vi "Parse Xml Recursively.vi"(6 "Map in":map{string, T1}(c390), 7 "Parent":string, 8 "error in":errorcluster, 9 "XML File Path":path, 10 "DOM document in":refnum<k20>, 11 "Tree Map in":refnum<class "Tree Map.lvclass">) -> (0 "error out":errorcluster, 2 "Map out":map{string, T1}(c390), 3 "Tree Map out":refnum<class "Tree Map.lvclass">)   [LabVIEW 2023, in "VI Properties Editor.lvlib"]
uses:
  VI Properties Editor.lvlib
  Tree Map/Tree Map/Tree Map.lvclass
  CTLs/XPath Get Attribute.ctl
  <vilib>/picture/picture.llb/imagedata.ctl
  CTLs/VI Properties.ctl
  CTLs/Control Properties.ctl
  CTLs/VI Data.ctl
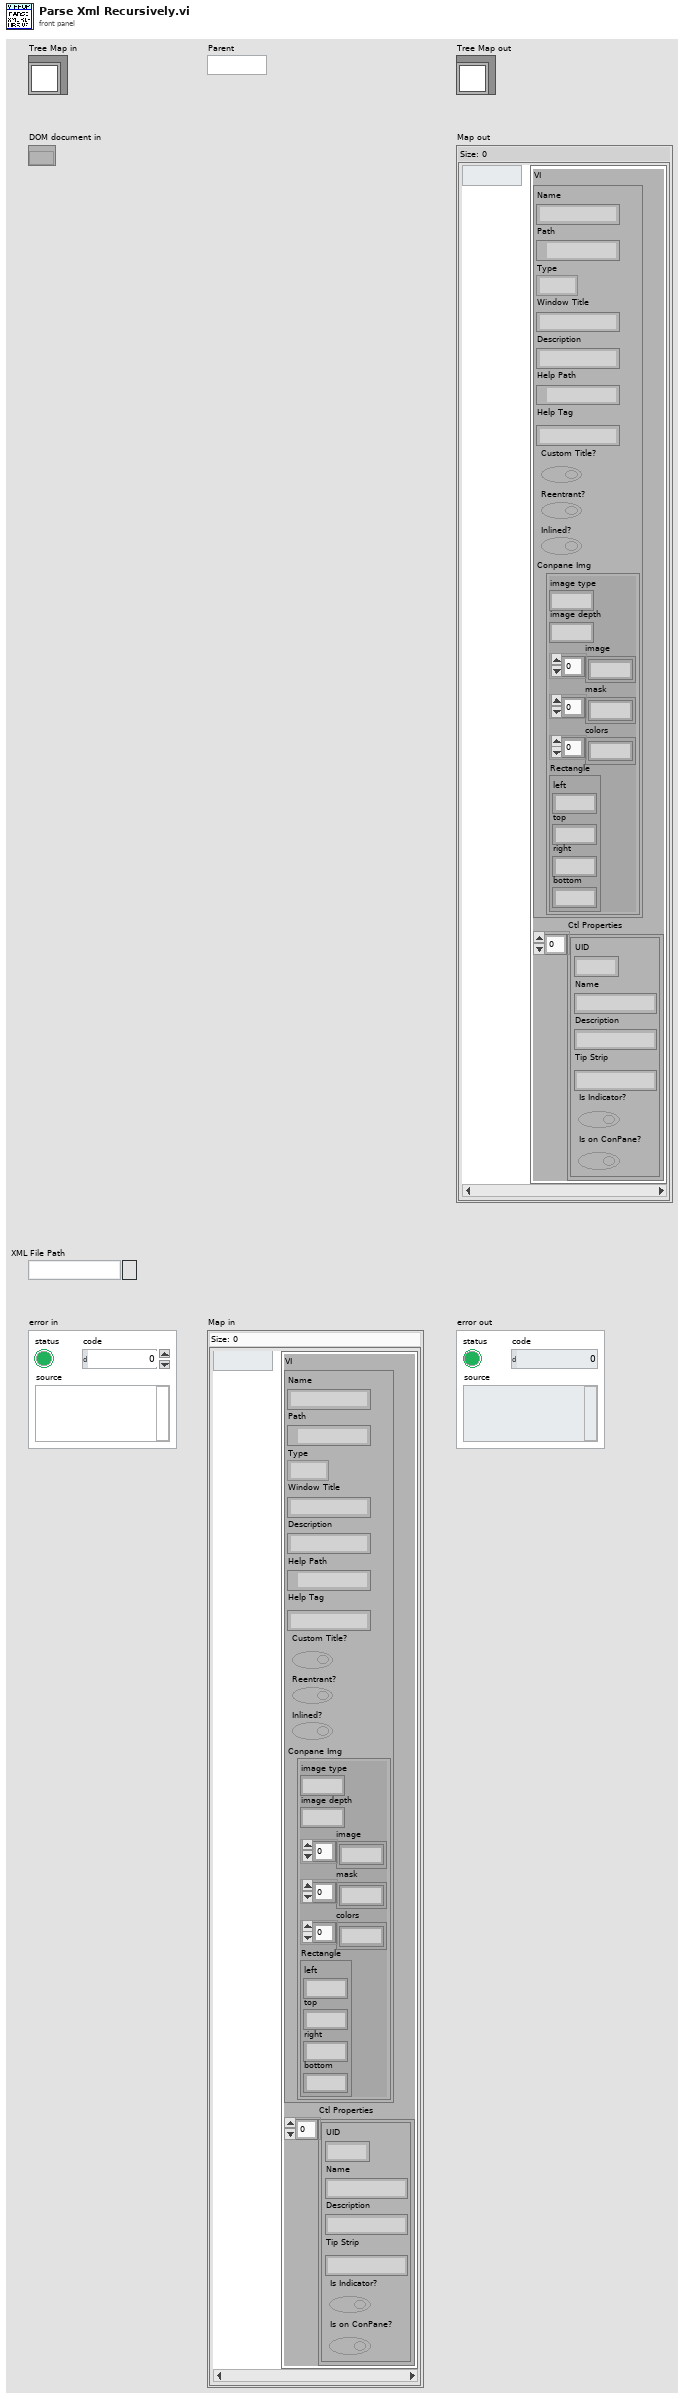
[diagram p1: front panel]
types:
  T1 = typedef "VI Properties Editor.lvlib/VI Data.ctl" = cluster{"VI":T2, "Ctl Properties":T4[]}
  T2 = typedef "VI Properties Editor.lvlib/VI Properties.ctl" = cluster{"Name":string, "Path":path, "Type":enum32{"invalid VI type", "Standard VI", "Control VI", "Global VI", "Polymorphic VI", "Configuration VI", "SubSystem", "Facade VI", "Method VI", "Statechart Diagram VI"}, "Window Title":string, "Description":string, "Help Path":path, "Help Tag":string, "Custom Title?":bool, "Reentrant?":bool, "Inlined?":bool, "Conpane Img":T3}
  T3 = typedef "imagedata.ctl" = cluster{"image type":i32, "image depth":i32, "image":u8[], "mask":u8[], "colors":u32[], "Rectangle":cluster{"left":i16, "top":i16, "right":i16, "bottom":i16}}
  T4 = typedef "VI Properties Editor.lvlib/Control Properties.ctl" = cluster{"UID":i32, "Name":string, "Description":string, "Tip Strip":string, "Is Indicator?":bool, "Is on ConPane?":bool}
  T5 = typedef "VI Properties Editor.lvlib/XPath Get Attribute.ctl" = enum16{"Item[@Type='VI']/@URL", "Item[@Type='LVClass']/@URL", "Item[@Type='Library']/@URL", "@Name"}
  T6 = typedef "VI Properties Editor.lvlib/VI Data Map.ctl" = map{string, cluster{"VI":T2, "Ctl Properties":T4[]}}
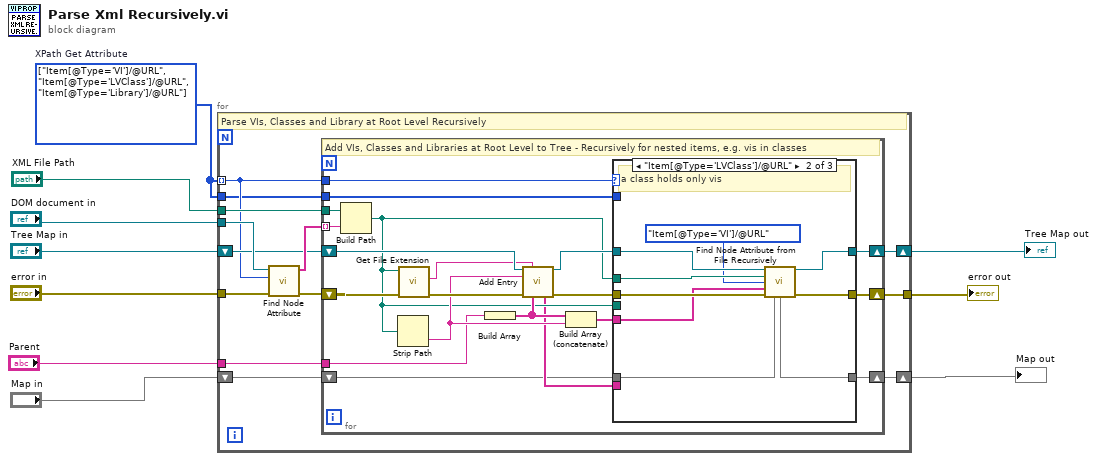
[diagram p0: block diagram]
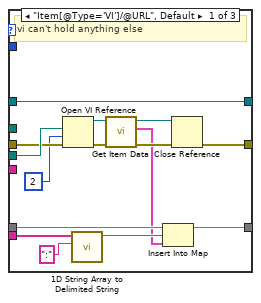
[diagram p2: hidden frame]
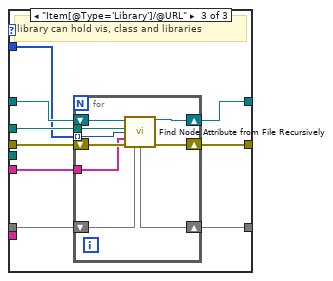
[diagram p3: hidden frame]
diagram:
  w4 = T5[] [enum."Item[@Type='VI']/@URL", enum."Item[@Type='LVClass']/@URL", enum."Item[@Type='Library']/@URL"] items=["Item[@Type='VI']/@URL", "Item[@Type='LVClass']/@URL", "Item[@Type='Library']/@URL", "@Name"]  # XPath Get Attribute
  n1 = for {
    tunnel: "XML File Path" -> [w22]
    tunnel: [w21] -> w6
    tunnel: "DOM document in" -> [w18]
    tunnel: "error in" -> [w17]
    shift-right: [w20] -> w7
    shift-left: "Tree Map in" -> [w16]
    tunnel: "Parent" -> [w15]
    shift-right: [w13] -> w5
    shift-left: "Map in" -> [w14]
    tunnel: w4 -> [w12] mode=indexing
    tunnel: w4 -> [w11]
    # "Parse VIs, Classes and Library at Root Level Recursively"
    n2 = call "Find Node Attribute.vi"("error in"=w17, "XPath"=w12, "Node"=w18) -> ("error out"=w19:errorcluster, "Attribute"=w23:string[])  [unwired: 7 in]
    n3 = for {
      shift-right: [w43] -> w21
      shift-left: w19 -> [w35]
      tunnel: w12 -> [w36]
      tunnel: w22 -> [w41]
      tunnel: w23 -> [w42] mode=indexing
      shift-right: [w40] -> w20
      shift-left: w16 -> [w38]
      tunnel: w15 -> [w29]
      shift-right: [w25] -> w13
      shift-left: w14 -> [w26]
      tunnel: w11 -> [w24]
      # "Add VIs, Classes and Libraries at Root Level to Tree - Recursively for nested items, e.g. vis in classes"
      n4 = Build Path(base path=w41, name or relative path=w42) -> (appended path=w28:path)
      n5 = Strip Path(path=w28) -> (name=w32:string)  [unwired: 1 out]
      n6 = call <vilib>:"Get File Extension.vi"("error in (no error)"=w35, "file"=w28) -> ("error out"=w34:errorcluster, "lowercase file extension"=w33:string)  [unwired: 5 in, 3 out]
      n7 = Build Array(w29) -> (w30:string[])
      n8 = call "Add Entry.vi"("Tree Map in"=w38, "Symbol"=w33, "Name"=w32, "error in"=w34, "Parent (None)"=w30) -> ("Tree Map out"=w37:refnum<class "Tree Map.lvclass">, "Hierarchy"=w27:string[], "error out"=w39:errorcluster)  [unwired: 8 in]
      n9 = Build Array (concatenate)(w30, w32) -> (w31:string[])
      n10 = case shown="\"Item[@Type='LVClass']/@URL\"" w36 {
        tunnel: [w52 w67 w75] -> w43
        tunnel: [w58 w66 w74] -> w40
        tunnel: w39 -> [w55 w65 w76]
        tunnel: w37 -> [w58 w64 w73]
        tunnel: w28 -> [_ w63 w72]
        tunnel: w31 -> [_ w61 w71]
        tunnel: w28 -> [w56 _ _]
        tunnel: w27 -> [w50 _ _]
        tunnel: w26 -> [w48 w60 w69]
        tunnel: [w45 w59 w68] -> w25
        tunnel: w24 -> [_ _ w70]
        frame "Item[@Type='VI']/@URL", Default {
          # "vi can't hold anything else"
          n11 = Open VI Reference(vi path=w56, options=2, error in (no error)=w55) -> (vi reference=w53:refnum<vi>, error out=w54:errorcluster)  [unwired: 3 in]
          n12 = call <vilib>:"1D String Array to Delimited String.vi"("delimiter"=":", "string array"=w50) -> ("delimited string"=w47:string)  [unwired: 9 in]
          n13 = call "Get Item Data.vi"("error in (no error)"=w54, "VI Ref"=w53) -> ("error out"=w57:errorcluster, "VI Data"=w46:T1, "VI Ref out"=w51:refnum<vi>)  [unwired: 7 in]
          n14 = Insert Into Map(map in=w48, key=w47, value=w46) -> (map out=w45:map{string, T1})  [unwired: 2 out]
          n15 = Close Reference(reference=w51, error in (no error)=w57) -> (error out=w52:errorcluster)
        }
        frame "Item[@Type='LVClass']/@URL" {
          # "a class holds only vis"
          n16 = call "Find Node Attribute from File Recursively.vi"("Tree Map in"=w64, "Path to XML document"=w63, "XPath"=XPath_Get_Attribute."Item[@Type='VI']/@URL", "Parent"=w61, "error in"=w65, "VI Data Map in"=w60) -> ("Tree Map out"=w66:refnum<class "Tree Map.lvclass">, "VI Data Map out"=w59:T6, "error out"=w67:errorcluster)  [unwired: 7 in]
        }
        frame "Item[@Type='Library']/@URL" {
          # "library can hold vis, class and libraries"
          n17 = for {
            tunnel: w72 -> [w81]
            tunnel: w70 -> [w80] mode=indexing
            tunnel: w71 -> [w79]
            shift-right: [w84] -> w75
            shift-left: w76 -> [w85]
            shift-right: [w83] -> w74
            shift-left: w73 -> [w82]
            shift-right: [w77] -> w68
            shift-left: w69 -> [w78]
            n18 = call "Find Node Attribute from File Recursively.vi"("Tree Map in"=w82, "Path to XML document"=w81, "XPath"=w80, "Parent"=w79, "error in"=w85, "VI Data Map in"=w78) -> ("Tree Map out"=w83:refnum<class "Tree Map.lvclass">, "VI Data Map out"=w77:T6, "error out"=w84:errorcluster)  [unwired: 7 in]
          }
        }
      }
    }
  }
  "Tree Map out" <- w7
  "error out" <- w6
  "Map out" <- w5
